vi "Write OCP_Mode.vi"(8 "error in":errorcluster, 10 "OCP Mode":T1, 11 "6700C in":refnum<class "6700C.lvclass">) -> (0 "error out":errorcluster, 3 "6700C out":refnum<class "6700C.lvclass">)   [LabVIEW 2019, in "6700C.lvlib" / "6700C.lvclass"]
uses:
  Library/6700C.lvclass
  builds/Instruments/PowerSupply.lvlibp/Custom Controls/OCP Mode.ctl
  builds/Instruments/PowerSupply.lvlibp/Library/PowerSupply.lvclass
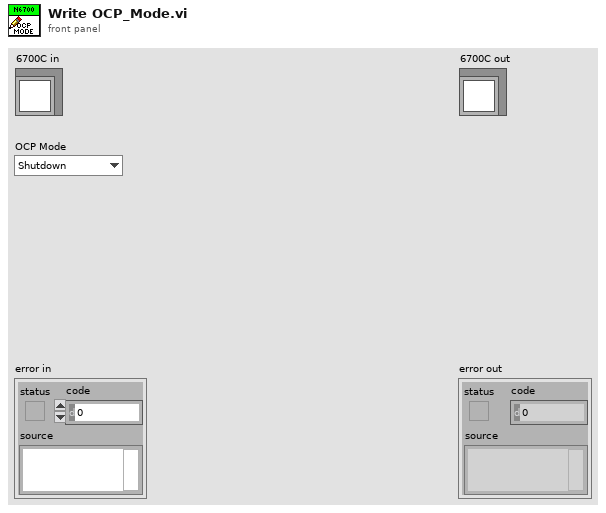
[diagram p1: front panel]
types:
  T1 = typedef "PowerSupply.lvlibp/PowerSupply.lvclass/OCP Mode.ctl" = enum16{"Shutdown", "Foldback"}
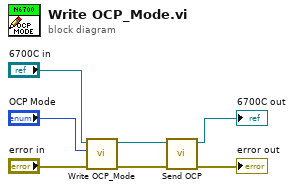
[diagram p0: block diagram]
diagram:
  n1 = call-parent "Write OCP_Mode.vi"("error in"="error in", "OCP Mode"="OCP Mode", "PowerSupply in"="6700C in") -> ("error out"=w3:errorcluster, "PowerSupply out"=w4:refnum<class "6700C.lvclass">)  [unwired: 7 in]
  n2 = call "Send OCP.vi"("error in"=w3, "6700C in"=w4) -> ("error out"=→"error out":errorcluster, "6700C out"=→"6700C out":refnum<class "6700C.lvclass">)  [unwired: 8 in]
